vi "LineToRect.vi"(0 "Lines":T1(array[cluster]), 1 "Margin of Error":i32=25) -> (2 "Good Lines":T1(array[cluster]))   [LabVIEW 2011]
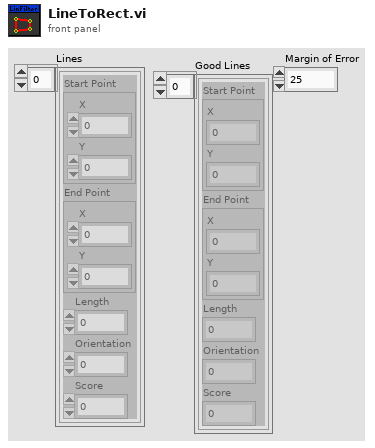
[diagram p1: front panel]
types:
  T1 = cluster{"Start Point":cluster{"X":sgl, "Y":sgl}, "End Point":cluster{"X":sgl, "Y":sgl}, "Length":dbl, "Orientation":dbl, "Score":dbl}[]
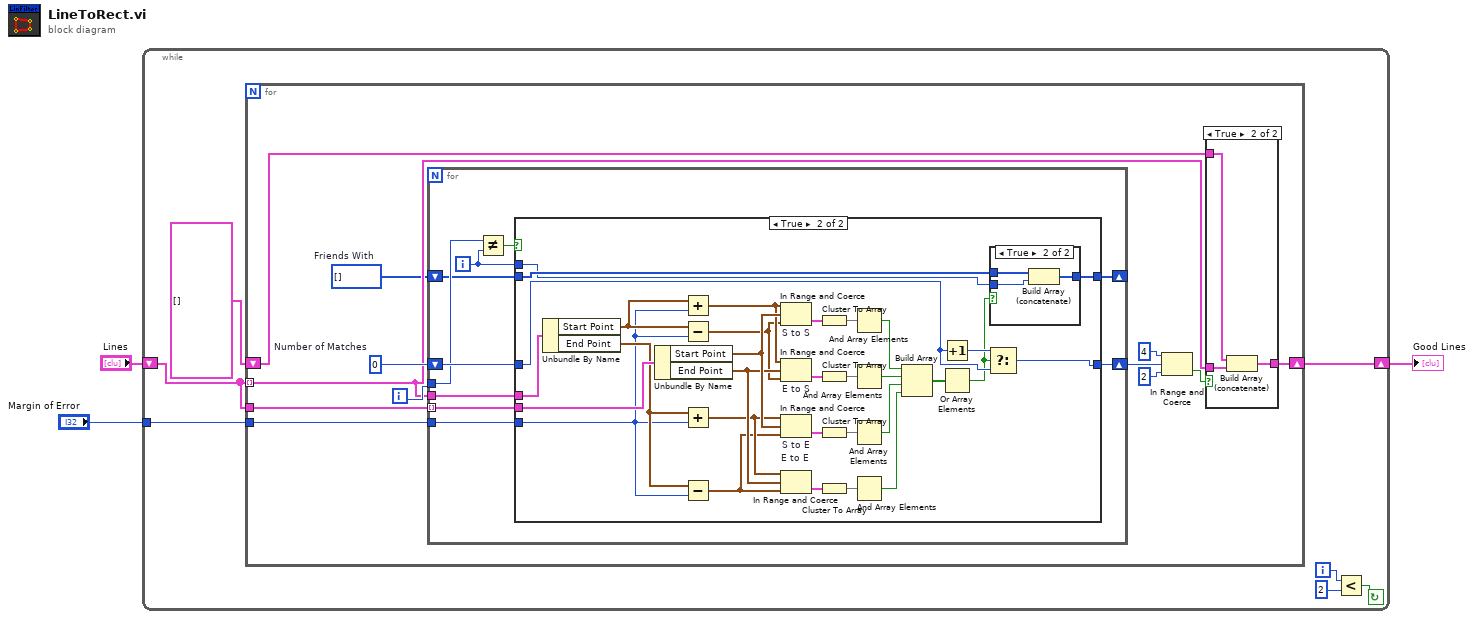
[diagram p0: block diagram]
diagram:
  n1 = while {
    shift-right: [w9] -> w3
    shift-left: "Lines" -> [w8]
    tunnel: "Margin of Error" -> [w4]
    i -> [w7]
    stop <- w6 continue-if-true
    n2 = for {
      tunnel: w8 -> [w13] mode=indexing
      tunnel: w8 -> [w22]
      shift-right: [w15] -> w9
      shift-left: T1 [] -> [w16]
      tunnel: w4 -> [w11]
      i -> [w20]
      w12 = i32[] []  # Friends With
      w21 = 0  # Number of Matches
      n3 = for {
        tunnel: w13 -> [w36]
        tunnel: w22 -> [w35] mode=indexing
        shift-right: [w33] -> w14
        shift-left: w21 -> [w34]
        tunnel: w20 -> [w32]
        shift-right: [w30] -> _
        shift-left: w12 -> [w29]
        tunnel: w11 -> [w27]
        i -> [w28]
        n4 = Not Equal?(x=w32, y=w28) -> (x != y?=w31:bool)
        n5 = case shown="True" w31 {
          tunnel: w36 -> [_ w69]
          tunnel: w35 -> [_ w68]
          tunnel: w34 -> [w38 w55]
          tunnel: [w38 w53] -> w33
          tunnel: [w37 w42] -> w30
          tunnel: w29 -> [w37 w41]
          tunnel: w28 -> [_ w40]
          tunnel: w27 -> [_ w39]
          frame False {
          }
          frame True {
            n6 = Unbundle By Name(w69) -> ("Start Point"=w65:cluster{"X":sgl, "Y":sgl}, "End Point"=w64:cluster{"X":sgl, "Y":sgl})
            n7 = Unbundle By Name(w68) -> ("Start Point"=w67:cluster{"X":sgl, "Y":sgl}, "End Point"=w66:cluster{"X":sgl, "Y":sgl})
            n8 = Add(x=w65, y=w39) -> (x+y=w63:cluster{"X":sgl, "Y":sgl})
            n9 = Subtract(x=w65, y=w39) -> (x-y=w62:cluster{"X":sgl, "Y":sgl})
            n10 = Add(x=w64, y=w39) -> (x+y=w61:cluster{"X":sgl, "Y":sgl})
            n11 = Subtract(x=w64, y=w39) -> (x-y=w60:cluster{"X":sgl, "Y":sgl})
            n12 = In Range and Coerce "S to S"(upper limit=w63, x=w67, lower limit=w62) -> (In Range?=w59:cluster{"X":bool, "Y":bool})  [unwired: 1 out]
            n13 = In Range and Coerce "E to S"(upper limit=w63, x=w66, lower limit=w62) -> (In Range?=w58:cluster{"X":bool, "Y":bool})  [unwired: 1 out]
            n14 = In Range and Coerce "S to E"(upper limit=w61, x=w67, lower limit=w60) -> (In Range?=w57:cluster{"X":bool, "Y":bool})  [unwired: 1 out]
            n15 = In Range and Coerce "E to E"(upper limit=w61, x=w66, lower limit=w60) -> (In Range?=w56:cluster{"X":bool, "Y":bool})  [unwired: 1 out]
            n16 = Cluster To Array(cluster=w59) -> (array=w52:bool[])
            n17 = Cluster To Array(cluster=w58) -> (array=w51:bool[])
            n18 = Cluster To Array(cluster=w57) -> (array=w50:bool[])
            n19 = Cluster To Array(cluster=w56) -> (array=w49:bool[])
            n20 = And Array Elements(Boolean array=w52) -> (logical AND=w47:bool)
            n21 = And Array Elements(Boolean array=w51) -> (logical AND=w46:bool)
            n22 = And Array Elements(Boolean array=w50) -> (logical AND=w45:bool)
            n23 = And Array Elements(Boolean array=w49) -> (logical AND=w44:bool)
            n24 = Build Array(w47, w46, w45, w44) -> (w48:bool[])
            n25 = Increment(x=w55) -> (x+1=w54:i32)
            n26 = Or Array Elements(Boolean array=w48) -> (logical OR=w43:bool)
            n27 = Select(t=w54, s=w43, f=w55) -> (s? t:f=w53:i32)
            n28 = case shown="True" w43 {
              tunnel: [w70 w72] -> w42
              tunnel: w41 -> [w70 w73]
              tunnel: w40 -> [_ w71]
              frame False {
              }
              frame True {
                n29 = Build Array (concatenate)(w73, w71) -> (w72:i32[])
              }
            }
          }
        }
      }
      n30 = In Range and Coerce(upper limit=4, x=w14, lower limit=2) -> (In Range?=w17:bool)  [unwired: 1 out]
      n31 = case shown="True" w17 {
        tunnel: w16 -> [w23 w26]
        tunnel: [w23 w24] -> w15
        tunnel: w13 -> [_ w25]
        frame False {
        }
        frame True {
          n32 = Build Array (concatenate)(w26, w25) -> (w24:T1)
        }
      }
    }
    n33 = Less?(x=w7, y=2) -> (x < y?=w6:bool)
  }
  "Good Lines" <- w3
